vi "VisualizeCHROMAOUT.vi"() -> ()   [LabVIEW 2018, in "Visualization.lvlib" / "VisualizeAcPwr.lvclass"]
doc: "This VI listens for any measurement data associated with the provided PluginName and displays it to the user for analysis. The display is only suitable for data coming from the Chroma Plugin."
uses:
  VisualizeAcPwr.lvclass
  VisualizeBase/VisualizeBase_class/Requests/VisUserEventType.ctl
  <vilib>/event_ctls.llb/usereventprio.ctl
  AcPwr/AcPwrShared/clMeasurmentData.ctl
  <extravilib>/ChannelInstances/Tag-bool/Read With Abort.vi
  <extravilib>/ChannelInstances/Tag-bool/Write With Abort.vi
  <extravilib>/ChannelInstances/Tag-bool/Instantiate.vi
  <extravilib>/ChannelInstances/Tag-bool/EndpointRead.vi
  <vilib>/Utility/error.llb/Error Cluster From Error Code.vi
  <extravilib>/ChannelInstances/Tag-bool/Endpoint.vi
  <vilib>/ErrorRing/Error Ring.xnode
  VisualizeBase/VisualizeBase_class/VisualizeBase.lvclass
  <userlib>/NIST/NISTErrorLib/NISTErrorLib.lvlib
  AcPwr/AcPwrShared/AcPwrShared.lvlib
  <extravilib>/ChannelInstances/Tag-bool.lvlib
panel:
  in  "Tab Control":enum32{"Chart", "XY Graph"}(tab)
  out "ChromaOutput":waveform(dbl)[](graph)=[{"t0"=timestamp(3657200531.6397257 s since 1904-01-01), "dt"=1.0, "Y"=[46.19]}, {"t0"=timestamp(3657200531.6397257 s since 1904-01-01), "dt"=1.0, "Y"=[2.0]}, {"t0"=timestamp(3657200531.6397257 s since 1904-01-01), "dt"=1.0, "Y"=[60.0]}]
  in  "PlotYAxis":u32[](array[numeric])=[0, 1, 0] max=1
  out "Incorrect DataType?":bool
  out "Chroma's Internal Errors/Warnings":string="No Error"
  out "Current (A)":dbl(knob) scale=0.0..15.0
  out "Voltage (V)":dbl(knob) scale=0.0..100.0
  out "XY Graph":cluster{dbl[], dbl[]}(graph)={[0.02, 0.02, 0.02, 0.02, 0.02, 0.02, 0.02, 0.02, 0.1, 0.1, 0.1, 0.1, 0.1, 0.11, 0.2, 0.2, 0.2, 0.2, 0.2, 0.2, 0.3, 0.3, 0.3, 0.3, 0.3, 0.3, 0.3, 0.37, 0.4, 0.4, 0.4, 0.4, 0.4, 0.4, 0.48, 0.5, 0.5, 0.5, 0.5, 0.5, 0.5, 0.59, 0.6, 0.6, 0.6, 0.6, 0.6, 0.6, 0.6, 0.69, 0.69, 0.69, 0.69, 0.69, 0.69, 0.71, 0.79, 0.79, 0.79, 0.79, 0.79, 0.79, 0.89, 0.89, 0.89, 0.89, 0.89, 0.89, 0.89, 1.0, 1.0, 1.0, 1.0, 1.0, 1.0, 1.0, 1.1, 1.1, 1.1, 1.09, 1.09, 1.09, 1.1, 1.19, 1.19, 1.2, 1.2, 1.2, 1.2, 1.2, 1.29, 1.29, 1.29, 1.29, 1.29, 1.29, 1.29, 1.39, 1.39, 1.39, 1.39, 1.39, 1.39, 1.39, 1.4, 1.49, 1.49, 1.49, 1.49, 1.49, 1.49, 1.57, 1.59, 1.59, 1.59, 1.59, 1.59, 1.59, 1.69, 1.69, 1.69, 1.69, 1.69, 1.69, 1.69, 1.79, 1.79, 1.79, 1.79, 1.79, 1.79, 1.79, 1.89, 1.89, 1.89, 1.89, 1.89, 1.89, 1.89, 1.99, 1.99, 1.99, 1.99, 1.99, 1.99, 2.0, 2.09, 2.09, 2.09, 2.09, 2.09, 2.09, 2.13, 2.19, 2.19, 2.19, 2.19, 2.19, 2.19, 2.29, 2.29, 2.29, 2.29, 2.29, 2.29, 2.29, 2.29, 2.39, 2.39, 2.39, 2.39, 2.39, 2.39, 2.39, 2.49, 2.49, 2.49, 2.49, 2.49, 2.49, 2.51, 2.59, 2.59, 2.59, 2.59, 2.59, 2.59, 2.69, 2.69, 2.69, 2.69, 2.69, 2.69, 2.69, 2.79, 2.79, 2.79, 2.79, 2.79, 2.79, 2.79, 2.81, 2.89, 2.89, 2.89, 2.89, 2.89, 2.89, 2.89, 2.99, 2.99, 2.99, 2.99, 2.99, 2.99, 3.0, 3.09, 3.09, 3.09, 3.09, 3.09, 3.09, 3.1, 3.19, 3.19, 3.19, 3.19, 3.19, 3.19, 3.29, 3.29, 3.29, 3.29, 3.29, 3.29, 3.29, 3.39, 3.39, 3.39, 3.39, 3.39, 3.39, 3.39, 3.39, 3.49, 3.49, 3.49, 3.49, 3.49, 3.49, 3.49, 3.5, 3.59, 3.59, 3.59, 3.59, 3.59, 3.59, 3.6, 3.69, 3.69, 3.69, 3.69, 3.69, 3.69, 3.79, 3.79, 3.79, 3.79, 3.79, 3.79, 3.79, 3.89, 3.89, 3.89, 3.89, 3.89, 3.89, 3.89, 3.99, 3.99, 3.99, 3.99, 3.99, 3.99, 3.99], [42.02, 41.83, 42.15, 41.98, 41.52, 41.47, 41.64, 41.55, 41.51, 41.49, 41.46, 41.51, 41.41, 41.39, 41.42, 41.42, 41.41, 41.4, 41.29, 41.3, 41.32, 41.33, 41.32, 41.31, 41.32, 41.21, 41.21, 41.2, 41.2, 41.21, 41.22, 41.21, 41.1, 41.1, 41.09, 41.1, 41.09, 41.11, 41.1, 40.98, 40.99, 40.98, 40.98, 40.99, 40.99, 40.98, 40.98, 40.86, 40.86, 40.88, 40.87, 40.88, 40.87, 40.87, 40.74, 40.75, 40.75, 40.75, 40.73, 40.76, 40.63, 40.63, 40.62, 40.64, 40.64, 40.61, 40.64, 40.6, 40.5, 40.46, 40.5, 40.51, 40.5, 40.51, 40.37, 40.37, 40.37, 40.37, 40.37, 40.38, 40.37, 40.36, 40.22, 40.23, 40.23, 40.24, 40.23, 40.24, 40.1, 40.09, 40.07, 40.11, 40.09, 40.09, 40.11, 39.96, 39.96, 39.95, 39.96, 39.96, 39.96, 39.94, 39.81, 39.79, 39.79, 39.81, 39.8, 39.79, 39.79, 39.81, 39.65, 39.65, 39.65, 39.65, 39.64, 39.64, 39.65, 39.48, 39.48, 39.48, 39.48, 39.47, 39.48, 39.31, 39.31, 39.3, 39.31, 39.32, 39.31, 39.31, 39.14, 39.13, 39.13, 39.14, 39.13, 39.14, 39.13, 38.95, 38.95, 38.95, 38.94, 38.95, 38.95, 38.95, 38.75, 38.75, 38.76, 38.76, 38.75, 38.75, 38.75, 38.56, 38.56, 38.56, 38.56, 38.56, 38.55, 38.34, 38.34, 38.34, 38.33, 38.33, 38.34, 38.34, 38.11, 38.11, 38.1, 38.11, 38.12, 38.1, 38.11, 38.11, 37.87, 37.86, 37.86, 37.88, 37.86, 37.88, 37.86, 37.6, 37.61, 37.61, 37.61, 37.61, 37.61, 37.62, 37.33, 37.34, 37.33, 37.34, 37.34, 37.34, 37.04, 37.04, 37.05, 37.04, 37.06, 37.05, 37.04, 36.72, 36.72, 36.71, 36.72, 36.73, 36.72, 36.71, 36.72, 36.38, 36.37, 36.39, 36.37, 36.37, 36.38, 36.37, 36.0, 36.0, 35.99, 36.0, 35.99, 36.0, 35.99, 35.59, 35.59, 35.58, 35.58, 35.58, 35.58, 35.12, 35.12, 35.12, 35.13, 35.13, 35.13, 35.12, 34.6, 34.59, 34.59, 34.59, 34.59, 34.59, 34.59, 34.6, 33.97, 33.97, 33.98, 33.97, 33.98, 33.98, 33.98, 33.26, 33.27, 33.26, 33.26, 33.26, 33.26, 33.26, 33.26, 32.38, 32.39, 32.39, 32.37, 32.37, 32.39, 32.38, 31.25, 31.24, 31.25, 31.25, 31.25, 31.25, 29.64, 29.66, 29.66, 29.67, 29.65, 29.66, 29.66, 27.14, 27.15, 27.15, 27.15, 27.14, 27.14, 27.15, 17.86, 17.84]}
  in  "PluginName":string="AcPwr.ChromaPowerSupply0"
  out "ErrorArray":errorcluster[](array[cluster])
  in  "btnStop":bool
  in  "btnReset":bool
  in  "btnClear":bool
  # "0=Left Axis and 1=Right Axis"
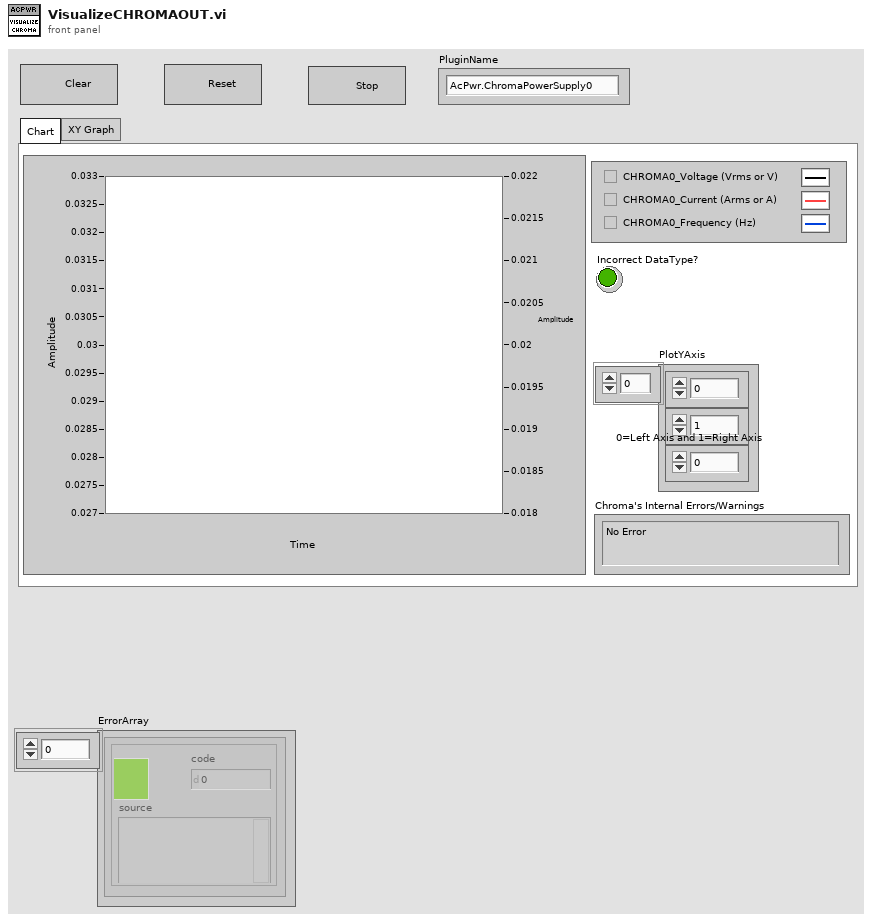
[diagram p1: front panel]
types:
  T1 = typedef "Visualization.lvlib/VisualizeBase.lvclass/VisRequestEvents.ctl" = cluster{"StopRequest":refnum<user-event>, "ResetRequest":refnum<user-event>, "FP Pop In or Out":refnum<user-event>}
  T2 = typedef "AcPwrShared.lvlib/AcPwrBroadcastEvents.ctl" = cluster{"DidInit":refnum<user-event>, "StatusUpdate":refnum<user-event>, "ErrorReport":refnum<user-event>, "DidStop":refnum<user-event>, "PathToINI":refnum<user-event>, "Measurements":refnum<user-event>, "LoadConfigFile":refnum<user-event>, "GetSettings":refnum<user-event>, "SetSettings":refnum<user-event>, "GetType&ID":refnum<user-event>, "GotSettings":refnum<user-event>}
  T3 = typedef "AcPwrShared.lvlib/clMeasurmentData.ctl" = cluster{"MeasName":string, "XML Data":string, "WaveformData":waveform(dbl)[]}
  T4 = typedef "Visualization.lvlib/VisualizeBase.lvclass/VisUserEventType.ctl" = cluster{"BusIndex":i8, "Data":variant}
  T5 = typedef "usereventprio.ctl" = enum32{"high priority", "normal priority"}
  T6 = typedef "Tag-bool.lvlib/))Channel.ctl" = refnum<queue>
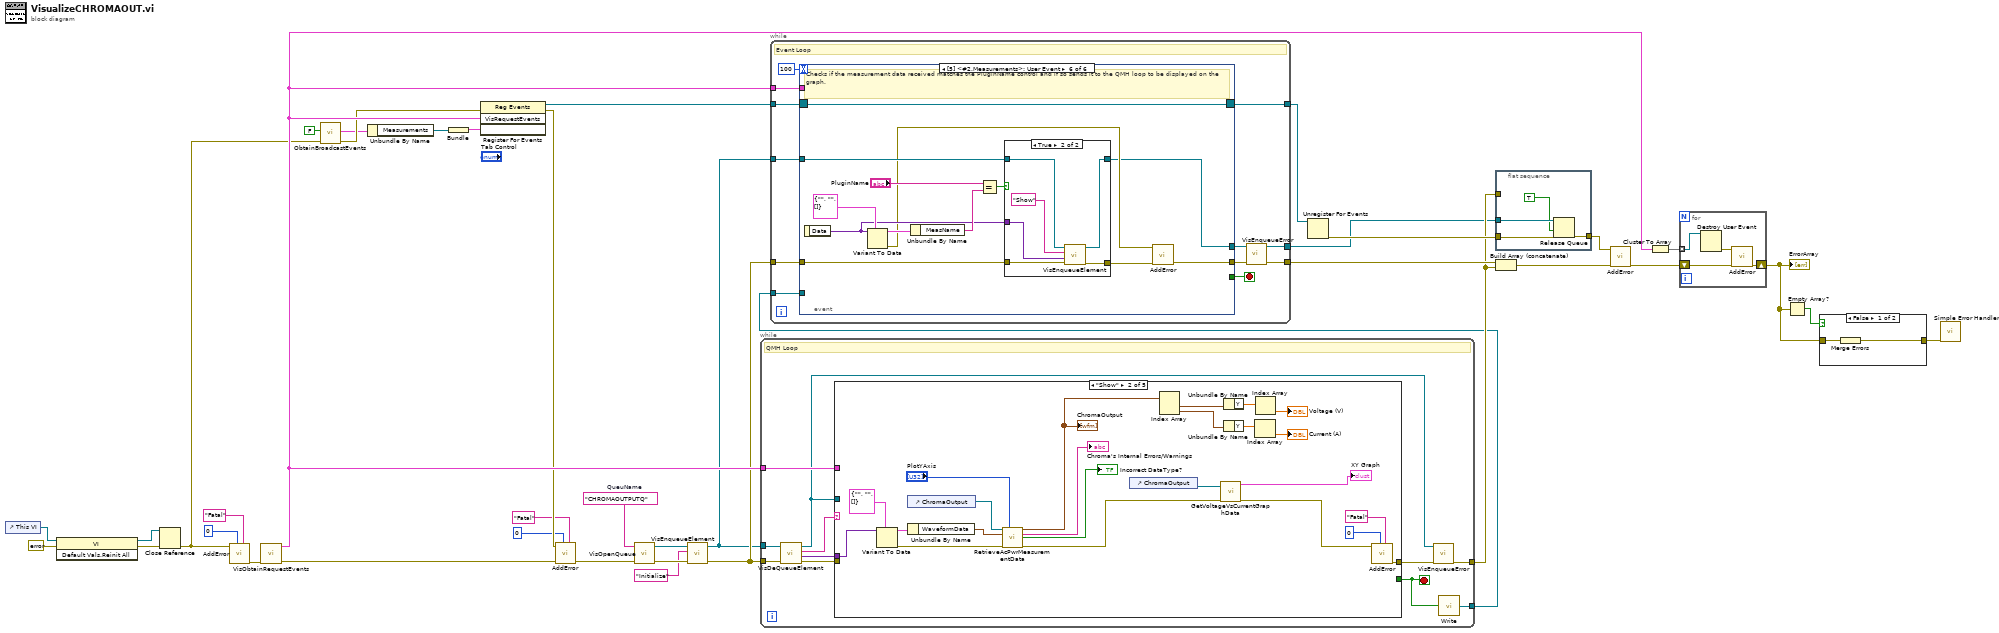
[diagram p0: block diagram]
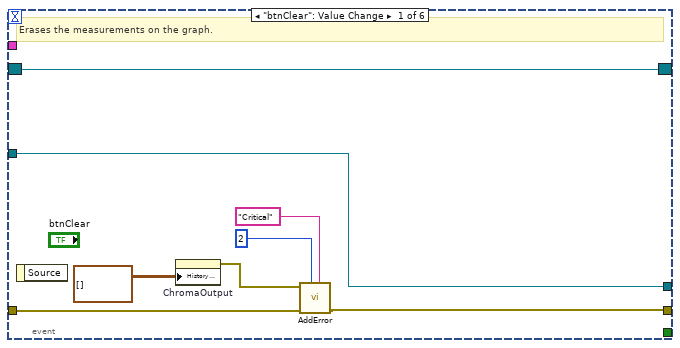
[diagram p2: hidden frame]
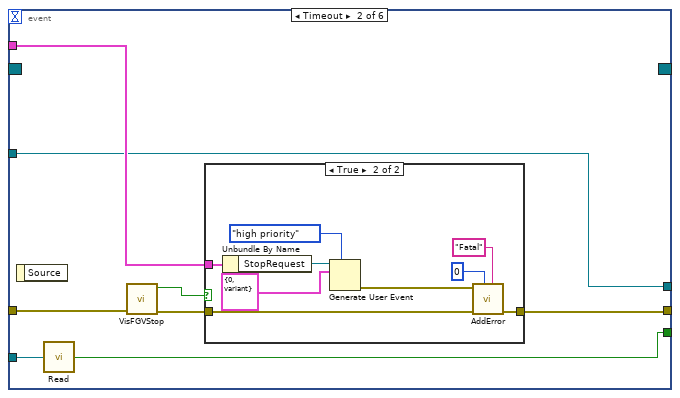
[diagram p3: hidden frame]
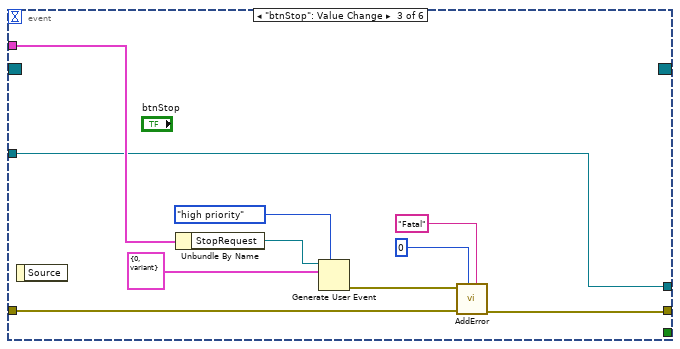
[diagram p5: hidden frame]
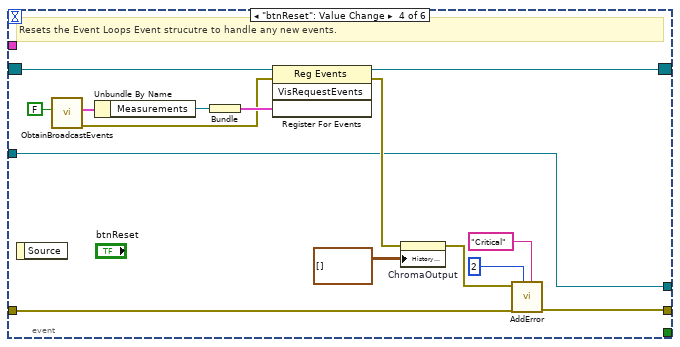
[diagram p6: hidden frame]
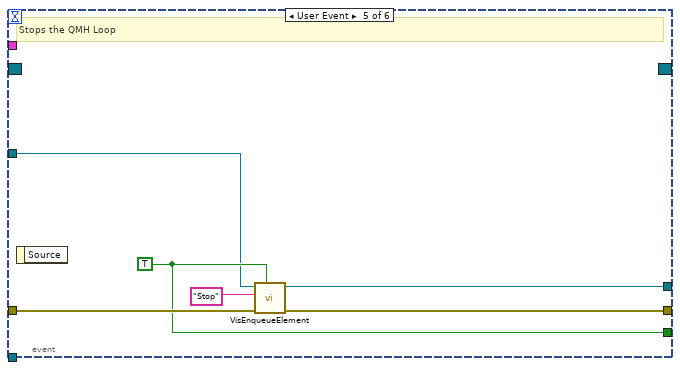
[diagram p7: hidden frame]
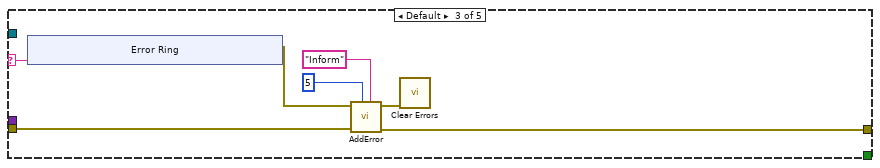
[diagram p10: hidden frame]
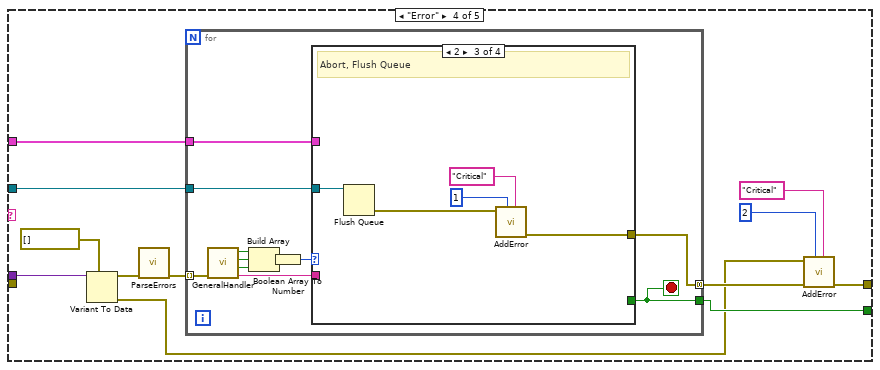
[diagram p11: hidden frame]
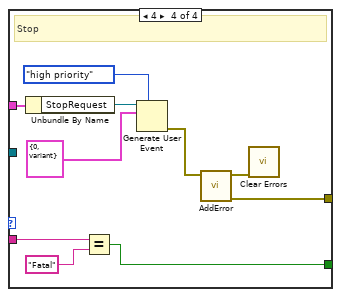
[diagram p14: hidden frame]
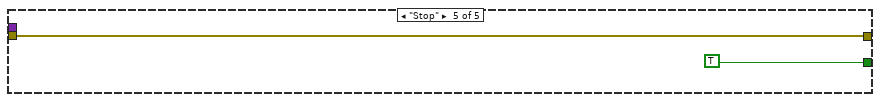
[diagram p15: hidden frame]
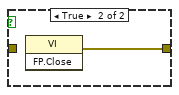
[diagram p16: hidden frame]
diagram:
  w10 = "CHROMAOUTPUTQ"  # QueuName
  n1 = control-ref of="This VI"() -> (w26:refnum<vi>)
  n2 = invoke class="VI" method="Default Vals.Reinit All"(reference=w26, error in=errorcluster {"status"=FALSE, "code"=0, "source"=""} ("error in (no error)")) -> (reference out=w23:refnum<vi>, error out=w24:errorcluster)  [unwired: 1 in, 1 out]
  n3 = Close Reference(reference=w23, error in (no error)=w24) -> (error out=w14:errorcluster)
  n4 = call <userlib>:"AddError.vi"("Severity"="Fatal", "Priority"=u8 0, "error in (no error)"=w14) -> ("ErrorArray Out"=w38:errorcluster[])  [unwired: 7 in, 1 out]
  n5 = call "VisObtainRequestEvents.vi"("Error"=w38) -> ("Error"=w21:errorcluster[], "VisRequestEvents"=w30:T1)  [unwired: 9 in]
  n6 = call "ObtainBroadcastEvents.vi"("error in (no error)"=w14, "CreateNew? (F)"=FALSE) -> ("error out"=w15:errorcluster, "clAcPwrEvents"=w13:T2)  [unwired: 8 in]
  n7 = Unbundle By Name(w13) -> ("Measurements"=w28:refnum<user-event>)
  n8 = Bundle("Measurements"=w28) -> (w27:cluster{"Measurements":refnum<user-event>})  [unwired: 1 in]
  n9 = register-events(error in=w15, w30, w27) -> (reference out=w39:refnum<event-registration>, error out=w19:errorcluster)  [unwired: 1 in]
  n10 = call <userlib>:"AddError.vi"("Severity"="Fatal", "Priority"=u8 0, "ErrorArray In"=w21, "error in (no error)"=w19) -> ("ErrorArray Out"=w11:errorcluster[])  [unwired: 6 in, 1 out]
  n11 = call "VisOpenQueue.vi"("Error Array In"=w11, "QueueName"=w10) -> ("Error Array Out"=w8:errorcluster[], "queue out"=w9:refnum<queue>)  [unwired: 8 in]
  n12 = call "VisEnqueueElement.vi"("Error Array In"=w8, "Message"="Initialize", "queue in"=w9) -> ("Error Array Out"=w6:errorcluster[], "queue out"=w5:refnum<queue>)  [unwired: 7 in]
  n13 = while {
    tunnel: w6 -> [w44]
    tunnel: [w47] -> w16
    tunnel: w5 -> [w43]
    tunnel: w30 -> [w49]
    tunnel: [w40] -> w1
    stop <- w50 stop-if-true
    # "QMH Loop"
    n14 = call "VisDeQueueElement.vi"("Error Array In"=w44, "Queue In"=w43) -> ("Error Array Out"=w42:errorcluster[], "Data"=w45:variant, "Message"=w46:string, "Queue Out"=w41:refnum<queue>)  [unwired: 6 in]
    n15 = case shown="\"Show\"" w46 {
      selector: w46 -> [_ _ w81 _ _]
      tunnel: w45 -> [_ w59 _ w100 _]
      tunnel: w42 -> [w51 _ w79 _ w127]
      tunnel: [w51 w74 w78 w90 w127] -> w48
      tunnel: [_ _ _ w96 TRUE] -> w50
      tunnel: w49 -> [_ _ _ w95 _]
      tunnel: w41 -> [_ _ _ w94 _]
      frame "Initialize" {
      }
      frame "Show" {
        n16 = Variant To Data(type=T3 {"MeasName"="", "XML Data"="", "WaveformData"=[]} ("MeasurmentDataCluster"), Variant=w59) -> (data=w57:T3, error out=w58:errorcluster)  [unwired: 1 in]
        n17 = control-ref of="ChromaOutput"() -> (w73:refnum<vi>)
        n18 = Unbundle By Name(w57) -> ("WaveformData"=w56:waveform(dbl)[])
        n19 = call "RetrieveAcPwrMeasurementData.vi"("WaveformChartReference"=w73, "PlotYScale"="PlotYAxis", "WaveformArrayIn"=w56, "error in (no error)"=w58) -> ("WaveformArrayOut"=w66:waveform(dbl)[], "OutputString(Chroma)"=→"Chroma's Internal Errors/Warnings":string, "Incorrect DataType?"=→"Incorrect DataType?":bool, "error out"=w68:errorcluster)  [unwired: 7 in, 1 out]
        "ChromaOutput" <- w66
        n20 = control-ref of="ChromaOutput"() -> (w52:refnum<vi>)
        n21 = Index Array(array=w66) -> (element #1=w65:waveform(dbl), element #2=w64:waveform(dbl))  [unwired: 2 in]
        n22 = call "GetVoltageVsCurrentGraphData.vi"("error in (no error)"=w68, "WaveformChart in"=w52) -> ("error out"=w54:errorcluster, "Cluster"=→"XY Graph":cluster{dbl[], dbl[]})  [unwired: 8 in]
        n23 = Unbundle By Name(w65) -> ("Y"=w63:dbl[])
        n24 = Unbundle By Name(w64) -> ("Y"=w62:dbl[])
        n25 = Index Array(array=w62) -> (element=→"Current (A)":dbl)  [unwired: 1 in]
        n26 = Index Array(array=w63) -> (element=→"Voltage (V)":dbl)  [unwired: 1 in]
        n27 = call <userlib>:"AddError.vi"("Severity"="Fatal" ("String"), "Priority"=u8 0, "error in (no error)"=w54) -> ("ErrorArray Out"=w74:errorcluster[])  [unwired: 7 in, 1 out]
      }
      frame Default {
        n28 = xnode "Error Ring"("parameter 0"=w81) -> ("error out"=w80:errorcluster)
        n29 = call <userlib>:"AddError.vi"("Severity"="Inform" ("String"), "Priority"=u8 5, "ErrorArray In"=w79, "error in (no error)"=w80) -> ("ErrorArray Out"=w78:errorcluster[], "error out"=w77:errorcluster)  [unwired: 6 in]
        n30 = call <vilib>:"Clear Errors.vi"("error in (no error)"=w77) -> ()  [unwired: 5 in, 2 out]
      }
      frame "Error" {
        n31 = Variant To Data(type=errorcluster[] [], Variant=w100) -> (data=w98:errorcluster[], error out=w89:errorcluster)  [unwired: 1 in]
        n32 = call <userlib>:"ParseErrors.vi"("ErrorArray"=w98) -> ("ErrorArray"=w97:errorcluster[])  [unwired: 8 in, 2 out]
        n33 = for {
          tunnel: w97 -> [w111] mode=indexing
          tunnel: [w105] -> w91 mode=concatenating
          tunnel: [w103] -> w96
          tunnel: w95 -> [w102]
          tunnel: w94 -> [w101]
          stop <- w103 stop-if-true
          n34 = call <userlib>:"GeneralHandler.vi"("error in (no error)"=w111) -> ("Severity"=w104:string, "Stop"=w108:bool, "Abort"=w109:bool, "Continue"=w110:bool)  [unwired: 6 in, 1 out]
          n35 = Build Array(w110, w109, w108) -> (w107:bool[])
          n36 = Boolean Array To Number(Boolean array=w107) -> (number=w106:u32)
          n37 = case shown="2" w106 {
            tunnel: [_ _ w116 w125] -> w105
            tunnel: w104 -> [_ _ _ w118]
            tunnel: [_ _ _ w120] -> w103
            tunnel: w102 -> [_ _ _ w119]
            tunnel: w101 -> [_ _ w112 _]
            frame 0, Default {
              # "No Dialog"
            }
            frame 1 {
              # "Continue"
            }
            frame 2 {
              # "Abort, Flush Queue"
              n38 = Flush Queue(queue=w112) -> (error out=w115:errorcluster)  [unwired: 1 in, 2 out]
              n39 = call <userlib>:"AddError.vi"("Severity"="Critical" ("String"), "Priority"=u8 1, "error in (no error)"=w115) -> ("ErrorArray Out"=w116:errorcluster[])  [unwired: 7 in, 1 out]
            }
            frame 4 {
              # "Stop"
              n40 = Unbundle By Name(w119) -> ("StopRequest"=w126:refnum<user-event>)
              n41 = Equal?(x=w118, y="Fatal" ("x")) -> (x = y?=w120:bool)
              n42 = Generate User Event(priority (normal)=usereventprio."high priority", user event=w126, event data cluster=T4 {"BusIndex"=0, "Data"=variant} ("event data")) -> (error out=w124:errorcluster)  [unwired: 1 in, 1 out]
              n43 = call <userlib>:"AddError.vi"("error in (no error)"=w124) -> ("ErrorArray Out"=w125:errorcluster[], "error out"=w121:errorcluster)  [unwired: 9 in]
              n44 = call <vilib>:"Clear Errors.vi"("error in (no error)"=w121) -> ()  [unwired: 5 in, 2 out]
            }
          }
        }
        n45 = call <userlib>:"AddError.vi"("Severity"="Critical", "Priority"=u8 2, "ErrorArray In"=w91, "error in (no error)"=w89) -> ("ErrorArray Out"=w90:errorcluster[])  [unwired: 6 in, 1 out]
      }
      frame "Stop" {
      }
    }
    n46 = call "VisEnqueueError.vi"("Error Array In"=w48, "Queue in"=w41) -> ("Error Array Out"=w47:errorcluster[])  [unwired: 8 in, 1 out]
    n47 = call <extravilib>:"Write.vi"("element"=w50) -> ("channel"=w40:T6)  [unwired: 1 out]
  }
  n48 = while {
    tunnel: w39 -> [w140]
    tunnel: [w134] -> w35
    tunnel: [w138] -> w37
    tunnel: w30 -> [w137]
    tunnel: w6 -> [w136]
    tunnel: w5 -> [w135]
    tunnel: [w131] -> w4
    tunnel: w1 -> [w129]
    stop <- w139 stop-if-true
    # "Event Loop"
    n49 = event shown="[5] <#2.Measurements>: User Event" {
      selector: w140 -> [w142 _ _ w191 _ w198]
      dyn-events: [w142 _ _ w190 _ w198] -> w138
      timeout: 100 -> [_ _ _ _ _ _]
      tunnel: [_ w149 _ _ w194 _] -> w139
      tunnel: [w145 w151 w173 w186 w196 w202] -> w133
      tunnel: w137 -> [_ w153 w175 _ _ _]
      tunnel: w136 -> [w146 w154 w176 w187 w197 w208]
      tunnel: w135 -> [w141 w152 w174 w177 w192 w210]
      tunnel: [w141 w152 w174 w177 w195 w199] -> w132
      tunnel: w129 -> [_ w150 _ _ _ _]
      event "btnClear": Value Change {
        # "Erases the measurements on the graph."
        n50 = event-data() -> ()  [unwired: 1 in, 1 out]
        n51 = property on="ChromaOutput" class="WFChart (strict)"("History Data"=waveform(dbl)[][] []) -> (error out=w144:errorcluster)  [unwired: 2 in, 1 out]
        n52 = call <userlib>:"AddError.vi"("Severity"="Critical", "Priority"=u8 2, "ErrorArray In"=w146, "error in (no error)"=w144) -> ("ErrorArray Out"=w145:errorcluster[])  [unwired: 6 in, 1 out]
      }
      event Timeout {
        n53 = event-data() -> ()  [unwired: 1 in, 1 out]
        n54 = call <extravilib>:"Read.vi"("channel"=w150) -> ("element"=w149:bool)  [unwired: 1 in, 1 out]
        n55 = call "VisFGVStop.vi"("Error In"=w154) -> ("Error Out"=w155:errorcluster[], "Value"=w156:bool)  [unwired: 9 in]
        n56 = case shown="True" w156 {
          tunnel: w155 -> [w157 w166]
          tunnel: [w157 w159] -> w151
          tunnel: w153 -> [_ w158]
          frame False {
          }
          frame True {
            n57 = Unbundle By Name(w158) -> ("StopRequest"=w164:refnum<user-event>)
            n58 = Generate User Event(priority (normal)=usereventprio."high priority", user event=w164, event data cluster=T4 {"BusIndex"=0, "Data"=variant} ("event data")) -> (error out=w165:errorcluster)  [unwired: 1 in, 1 out]
            n59 = call <userlib>:"AddError.vi"("Severity"="Fatal" ("String"), "Priority"=u8 0, "ErrorArray In"=w166, "error in (no error)"=w165) -> ("ErrorArray Out"=w159:errorcluster[])  [unwired: 6 in, 1 out]
          }
        }
      }
      event "btnStop": Value Change {
        n60 = event-data() -> ()  [unwired: 1 in, 1 out]
        n61 = Unbundle By Name(w175) -> ("StopRequest"=w171:refnum<user-event>)
        n62 = Generate User Event(priority (normal)=usereventprio."high priority", user event=w171, event data cluster=T4 {"BusIndex"=0, "Data"=variant} ("event data")) -> (error out=w172:errorcluster)  [unwired: 1 in, 1 out]
        n63 = call <userlib>:"AddError.vi"("Severity"="Fatal" ("String"), "Priority"=u8 0, "ErrorArray In"=w176, "error in (no error)"=w172) -> ("ErrorArray Out"=w173:errorcluster[])  [unwired: 6 in, 1 out]
      }
      event "btnReset": Value Change {
        # "Resets the Event Loops Event strucutre to handle any new events."
        n64 = event-data() -> ()  [unwired: 1 in, 1 out]
        n65 = call "ObtainBroadcastEvents.vi"("CreateNew? (F)"=FALSE) -> ("error out"=w180:errorcluster, "clAcPwrEvents"=w179:T2)  [unwired: 9 in]
        n66 = Unbundle By Name(w179) -> ("Measurements"=w189:refnum<user-event>)
        n67 = Bundle("Measurements"=w189) -> (w188:cluster{"Measurements":refnum<user-event>})  [unwired: 1 in]
        n68 = register-events(reference=w191, error in=w180, w188) -> (reference out=w190:refnum<event-registration>, error out=w182:errorcluster)  [unwired: 1 in]
        n69 = property on="ChromaOutput" class="WFChart (strict)"(error in=w182, "History Data"=waveform(dbl)[][] []) -> (error out=w181:errorcluster)  [unwired: 1 in, 1 out]
        n70 = call <userlib>:"AddError.vi"("Severity"="Critical", "Priority"=u8 2, "ErrorArray In"=w187, "error in (no error)"=w181) -> ("ErrorArray Out"=w186:errorcluster[])  [unwired: 6 in, 1 out]
      }
      event User Event {
        w194 = TRUE ("Priority? (F)")
        # "Stops the QMH Loop"
        n71 = event-data() -> ()  [unwired: 1 in, 1 out]
        n72 = call "VisEnqueueElement.vi"("Priority? (F)"=w194, "Error Array In"=w197, "Message"="Stop", "queue in"=w192) -> ("Error Array Out"=w196:errorcluster[], "queue out"=w195:refnum<queue>)  [unwired: 6 in]
      }
      event User Event {
        # "Checks if the measurement data received matches the PluginName control and if so sends it to the QMH loop to be displayed on the graph."
        n73 = event-data() -> ("Data"=w203:variant)  [unwired: 1 in]
        n74 = Variant To Data(type=T3 {"MeasName"="", "XML Data"="", "WaveformData"=[]} ("MeasurmentDataCluster"), Variant=w203) -> (data=w205:T3, error out=w200:errorcluster)  [unwired: 1 in]
        n75 = Unbundle By Name(w205) -> ("MeasName"=w204:string)
        n76 = Equal?(x="PluginName", y=w204) -> (x = y?=w209:bool)
        n77 = case shown="True" w209 {
          tunnel: [w211 w217] -> w201
          tunnel: w210 -> [w212 w216]
          tunnel: w208 -> [w211 w218]
          tunnel: [w212 w214] -> w199
          tunnel: w203 -> [_ w215]
          frame False {
          }
          frame True {
            n78 = call "VisEnqueueElement.vi"("Error Array In"=w218, "Data"=w215, "Message"="Show", "queue in"=w216) -> ("Error Array Out"=w217:errorcluster[], "queue out"=w214:refnum<queue>)  [unwired: 6 in]
          }
        }
        n79 = call <userlib>:"AddError.vi"("ErrorArray In"=w201, "error in (no error)"=w200) -> ("ErrorArray Out"=w202:errorcluster[])  [unwired: 8 in, 1 out]
      }
    }
    n80 = call "VisEnqueueError.vi"("Error Array In"=w133, "Queue in"=w132) -> ("Error Array Out"=w134:errorcluster[], "Queue out"=w131:refnum<queue>)  [unwired: 8 in]
  }
  n81 = Unregister For Events(event registration refnum=w37) -> (error out=w34:errorcluster)  [unwired: 1 in]
  n82 = flat-sequence {
    tunnel: w34 -> [w222]
    tunnel: [w221] -> w32
    tunnel: w4 -> [w220]
    tunnel: w16 -> [_]
    frame #0 {
      n83 = Release Queue(queue=w220, force destroy? (F)=TRUE, error in (no error)=w222) -> (error out=w221:errorcluster)  [unwired: 2 out]
    }
  }
  n84 = Build Array (concatenate)(w35, w16) -> (w33:errorcluster[])
  n85 = call <userlib>:"AddError.vi"("ErrorArray In"=w33, "error in (no error)"=w32) -> ("ErrorArray Out"=w31:errorcluster[])  [unwired: 8 in, 1 out]
  n86 = Cluster To Array(cluster=w30) -> (array=w36:refnum<user-event>[])
  n87 = for {
    tunnel: w36 -> [w226] mode=indexing
    shift-right: [w225] -> w3
    shift-left: w31 -> [w224]
    n88 = Destroy User Event(user event=w226) -> (error out=w223:errorcluster)  [unwired: 1 in]
    n89 = call <userlib>:"AddError.vi"("ErrorArray In"=w224, "error in (no error)"=w223) -> ("ErrorArray Out"=w225:errorcluster[])  [unwired: 8 in, 1 out]
  }
  "ErrorArray" <- w3
  n90 = Empty Array?(array=w3) -> (empty?=w29:bool)
  n91 = case shown="False" w29 {
    tunnel: [w227 w229] -> w2
    tunnel: w3 -> [w228 _]
    frame False {
      n92 = Merge Errors(w228) -> (w227:errorcluster)
    }
    frame True {
      n93 = invoke class="VI" method="FP.Close"() -> (error out=w229:errorcluster)  [unwired: 3 in, 2 out]
    }
  }
  n94 = call <vilib>:"Simple Error Handler.vi"("error in (no error)"=w2) -> ()  [unwired: 4 in, 5 out]
